vi "CommandBSTwCRC16.vi"() -> ()   [LabVIEW 2013]
uses:
  <vilib>/Utility/file.llb/Write To Spreadsheet File (I64).vi
panel:
  out "CRC =":u16 format="%x"
  out "Time stamps":timestamp[](array[timestamp])
  in  "file path (dialog if empty)":path
  in  "Tab Control":enum32{"Page 1", "Page 2"}(tab)
  in  "K":u8
  in  "R":u8
  in  "-":u8
  in  "1":i32
  in  "N Data Size":u16
  in  "Boolean":bool
  out "Packet":dbl[](array[numeric])
  out "Array":u8[](array[numeric])
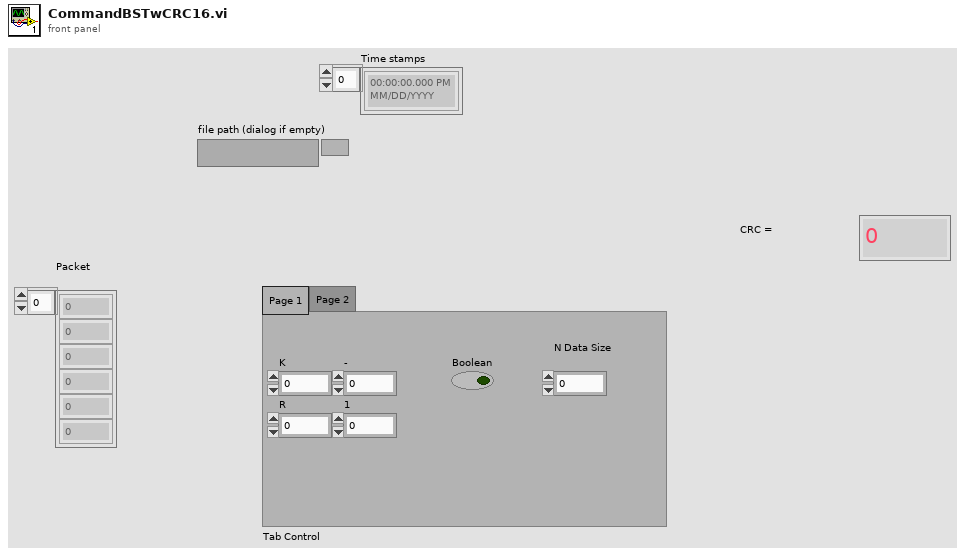
[diagram p1: front panel]
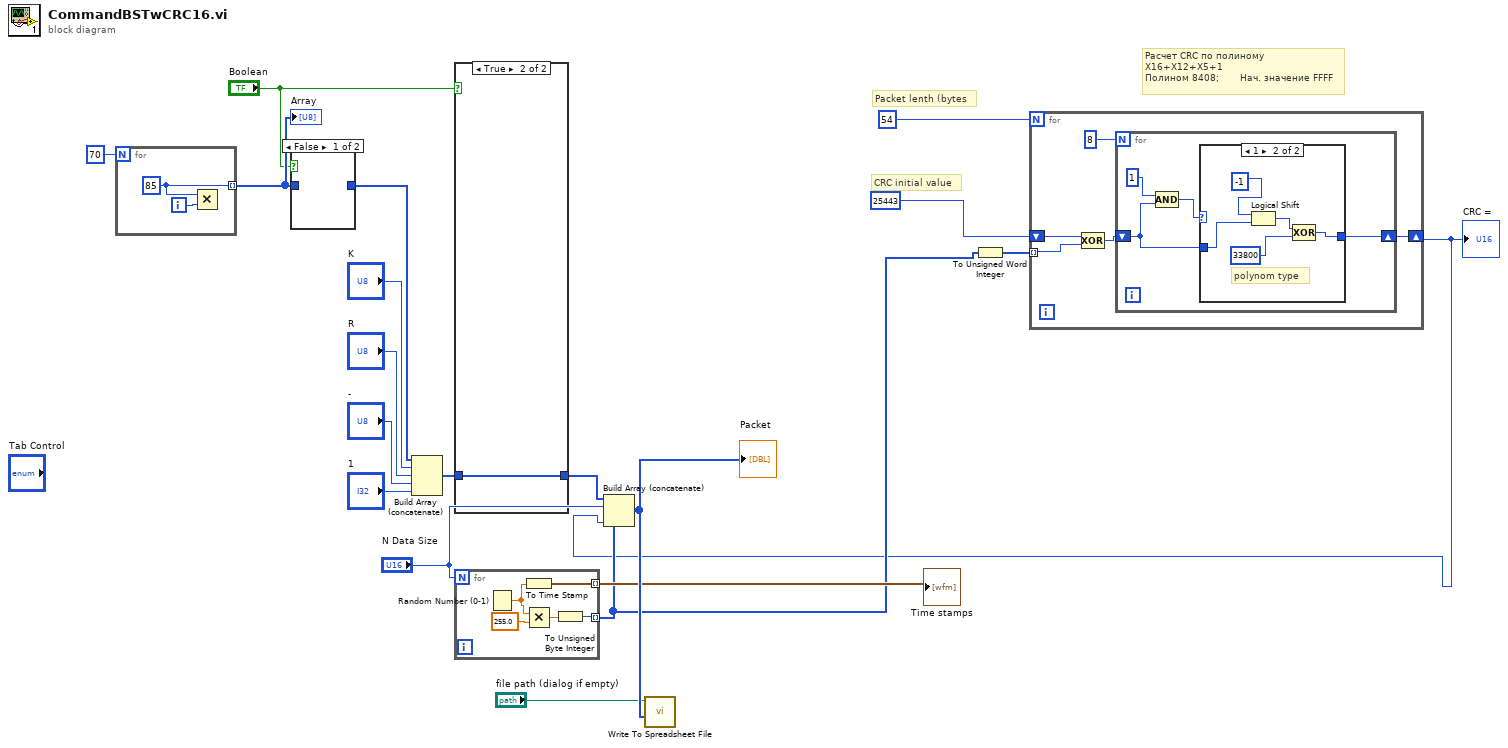
[diagram p0: block diagram]
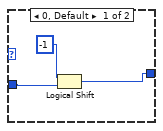
[diagram p2: hidden frame]
diagram:
  # "Packet lenth (bytes"
  # "CRC initial value"
  # "Расчет CRC по полиному X16+X12+X5+1\nПолином 8408;       Нач. значение FFFF"
  n1 = for {
    N: 70 -> [_]
    tunnel: [w20] -> w18 mode=indexing
    i -> [w21]
    w20 = 85 ("x")
    n2 = Multiply(x=w20, y=w21) -> ()  [unwired: 1 out]
  }
  "Array" <- w18
  n3 = case shown="False" "Boolean" {
    tunnel: w18 -> [_ w22]
    tunnel: [_ w22] -> w12
    frame False {
    }
    frame True {
    }
  }
  n4 = Build Array (concatenate)(w12, "K", "R", "-", "1") -> (w9:i32[])
  n5 = case shown="True" "Boolean" {
    tunnel: [_ w23] -> w11
    tunnel: w9 -> [_ w23]
    frame False {
    }
    frame True {
    }
  }
  n6 = for {
    N: "N Data Size" -> [_]
    tunnel: [w24] -> w2 mode=indexing
    tunnel: [w26] -> w6 mode=indexing
    n7 = Random Number (0-1)() -> (number: 0 to 1=w27:dbl)
    n8 = To Time Stamp(1:w27) -> (0:w26:timestamp)
    n9 = Multiply(x=w27, y=255.0) -> (x*y=w25:dbl)
    n10 = To Unsigned Byte Integer(number=w25) -> (unsigned 8bit integer=w24:u8)
  }
  "Time stamps" <- w6
  n11 = To Unsigned Word Integer(number=w2) -> (unsigned 16bit integer=w3:u16[])
  n12 = for {
    N: 54 -> [_]
    shift-right: [w30] -> w1
    shift-left: u16 25443 -> [w31]
    tunnel: w3 -> [w29] mode=indexing
    n13 = Compound Arithmetic op=XOR(w31, w29) -> (w32:u32)
    n14 = for {
      N: 8 -> [_]
      shift-right: [w36] -> w30
      shift-left: w32 -> [w35]
      n15 = Compound Arithmetic op=AND(u16 1, w35) -> (w34:u32)
      n16 = case shown="1" w34 {
        tunnel: [w39 w44] -> w36
        tunnel: w35 -> [w38 w41]
        frame 0, Default {
          n17 = Logical Shift(y=i16 -1, x=w38) -> (x << y=w39:u32)
        }
        frame 1 {
          # "polynom type"
          n18 = Logical Shift(y=i16 -1, x=w41) -> (x << y=w43:u32)
          n19 = Compound Arithmetic op=XOR(w43, u32 33800) -> (w44:u32)
        }
      }
    }
  }
  "CRC =" <- w1
  n20 = Build Array (concatenate)(w11, "N Data Size", w2, w1) -> (w8:u32[])
  "Packet" <- w8
  n21 = call-poly <vilib>:"Write To Spreadsheet File.vi"("1D data"=w8, "file path (dialog if empty)"="file path (dialog if empty)") -> ()  [unwired: 6 in, 1 out]
